vi "GV pixel clock change.vi"() -> ()   [LabVIEW 2017]
panel:
  out "Pixel clock change":bool
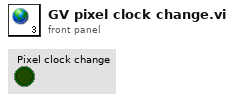
[diagram p1: front panel]
diagram:
